vi "Resize Parent FP to Largest Decoration - Drop In.vi"(8 "error in (no error)":errorcluster) -> (0 "error out":errorcluster)   [LabVIEW 2011]
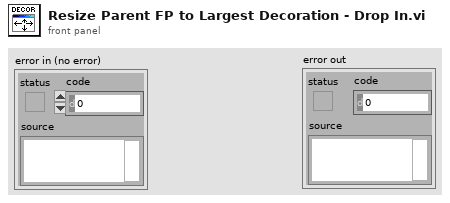
[diagram p1: front panel]
types:
  T1 = typedef "LVPositionTypeDef.ctl" = cluster{"Left":i32, "Top":i32}
  T2 = typedef "LVRectTypeDef.ctl" = cluster{"left":i16, "top":i16, "right":i16, "bottom":i16}
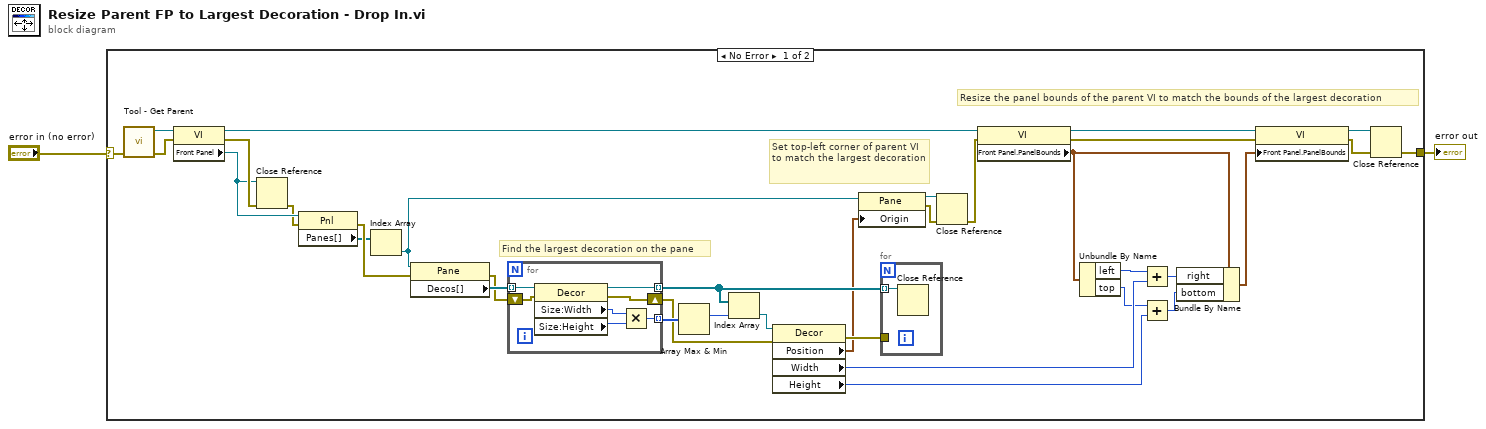
[diagram p0: block diagram]
diagram:
  n1 = case shown="No Error" "error in (no error)" {
    selector: "error in (no error)" -> [w6 w46]
    tunnel: [w3 w46] -> w1
    frame No Error {
      # "Resize the panel bounds of the parent VI to match the bounds of the largest decoration"
      # "Set top-left corner of parent VI to match the largest decoration"
      # "Find the largest decoration on the pane"
      n2 = call "Tool - Get Parent.vi"("error in (no error)"=w6) -> ("VI Refnum"=w37:refnum<vi>, "error out"=w36:errorcluster)  [unwired: 16 in, 1 out]
      n3 = property class="VI"(reference=w37, error in=w36) -> (reference out=w20:refnum<vi>, error out=w27:errorcluster, "Front Panel"=w26:refnum<vi>)
      n4 = Close Reference(reference=w26, error in (no error)=w27) -> (error out=w25:errorcluster)
      n5 = property class="Pnl"(reference=w26, error in=w25) -> (error out=w8:errorcluster, "Panes[]"=w7:refnum<vi>[])  [unwired: 1 out]
      n6 = Index Array(array=w7) -> (element=w21:refnum<vi>)  [unwired: 1 in]
      n7 = property class="Pane"(reference=w21, error in=w8) -> (error out=w34:errorcluster, "Decos[]"=w35:refnum<vi>[])  [unwired: 1 out]
      n8 = for {
        tunnel: w35 -> [w45] mode=indexing
        shift-right: [w40] -> w29
        shift-left: w34 -> [w44]
        tunnel: [w41] -> w33 mode=indexing
        tunnel: [w39] -> w30 mode=indexing
        n9 = property class="Decor"(reference=w45, error in=w44) -> (reference out=w39:refnum<vi>, error out=w40:errorcluster, "Size:Width"=w43:u32, "Size:Height"=w42:u32)
        n10 = Multiply(x=w43, y=w42) -> (x*y=w41:u32)
      }
      n11 = Array Max & Min(array=w33) -> (max index (indices)=w32:i32)  [unwired: 3 out]
      n12 = Index Array(array=w30, index=w32) -> (element=w31:refnum<vi>)
      n13 = property class="Decor"(reference=w31, error in=w29) -> (error out=w28:errorcluster, "Position"=w22:T1, "Width"=w16:u32, "Height"=w13:u32)  [unwired: 1 out]
      n14 = property class="Pane"(reference=w21, "Origin"=w22) -> (reference out=w23:refnum<vi>, error out=w24:errorcluster)  [unwired: 1 in]
      n15 = for {
        tunnel: w30 -> [w38] mode=indexing
        tunnel: w28 -> [_]
        n16 = Close Reference(reference=w38) -> ()  [unwired: 1 in, 1 out]
      }
      n17 = Close Reference(reference=w23, error in (no error)=w24) -> (error out=w19:errorcluster)
      n18 = property class="VI"(reference=w20, error in=w19) -> (reference out=w11:refnum<vi>, error out=w10:errorcluster, "Front Panel.PanelBounds"=w18:T2)
      n19 = Unbundle By Name(w18) -> ("left"=w17:i16, "top"=w14:i16)
      n20 = Add(x=w17, y=w16) -> (x+y=w15:u32)
      n21 = Add(x=w14, y=w13) -> (x+y=w12:u32)
      n22 = Bundle By Name(cluster=w18, "right"=w15, "bottom"=w12) -> (w9:T2)
      n23 = property class="VI"(reference=w11, error in=w10, "Front Panel.PanelBounds"=w9) -> (reference out=w5:refnum<vi>, error out=w4:errorcluster)
      n24 = Close Reference(reference=w5, error in (no error)=w4) -> (error out=w3:errorcluster)
    }
    frame Error {
    }
  }
  "error out" <- w1
